vi "relay_test.vi"() -> ()   [LabVIEW 2010]
panel:
  out "Acid Pump":bool
  out "error out":errorcluster
  in  "Action":u8(ring) items=["open dump on"=8, "pump acid on"=9, "air flush on"=10, "stop gas flow on"=11, "open dump off"=0, "pump acid off"=1, "air flush on"=2, "stop gas flow on"=3, "OpenAll"=30, "CloseAll"=29]
  in  "send relay action":bool
  out "Stop Gas Flow":bool
  out "Airflush":bool
  out "Dump":bool
  in  "stop":bool
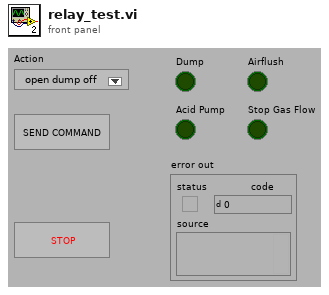
[diagram p1: front panel]
types:
  T1 = cluster{"VISA resource out":refnum<visa-resource-name>, "error out":errorcluster}
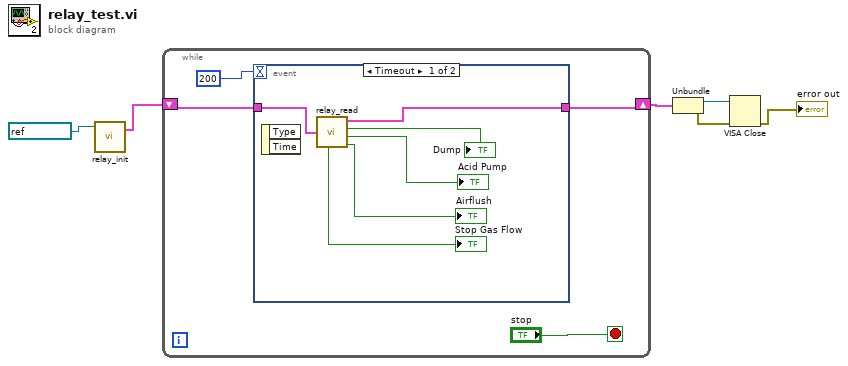
[diagram p0: block diagram]
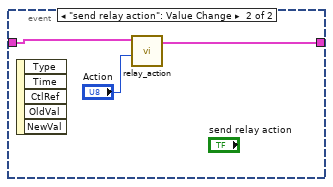
[diagram p2: hidden frame]
diagram:
  n1 = call "relay_init.vi"("VISA resource in"=refnum<visa-resource-name> "COM12" ("VISA resource out")) -> ("relay session out"=w5:T1)  [unwired: 3 in]
  n2 = while {
    shift-right: [w9] -> w4
    shift-left: w5 -> [w8]
    stop <- "stop" stop-if-true
    n3 = event shown="[0] Timeout" {
      selector: _ -> [_ _]
      dyn-events: _ -> [_ _]
      timeout: 200 -> [_ _]
      tunnel: [w16 w18] -> w9
      tunnel: w8 -> [w15 w19]
      event Timeout {
        n4 = event-data() -> ()  [unwired: 1 in, 2 out]
        n5 = call "relay_read.vi"("relay session in"=w15) -> ("Stop Gas Flow"=→"Stop Gas Flow":bool, "relay session out"=w16:T1, "Dump"=→"Dump":bool, "Acid Pump"=→"Acid Pump":bool, "Airflush"=→"Airflush":bool)  [unwired: 3 in]
      }
      event "send relay action": Value Change {
        n6 = event-data() -> ()  [unwired: 1 in, 5 out]
        n7 = call "relay_action.vi"("relay session in"=w19, "Action"="Action") -> ("relay session out"=w18:T1)  [unwired: 6 in]
      }
    }
  }
  n8 = Unbundle(w4) -> ("VISA resource out"=w3:refnum<visa-resource-name>, "error out"=w2:errorcluster)
  n9 = VISA Close(VISA resource name=w3, error in (no error)=w2) -> (error out=→"error out":errorcluster)
